vi "UUDT Engine.vi"() -> ()   [LabVIEW 2013, in "GMLAN.lvlib"]
uses:
  GMLAN.lvlib
  <vilib>/Automotive Diagnostic Command Set/Diagnostic Transport.llb/Diag Reference.ctl
  <vilib>/Automotive Diagnostic Command Set/Diagnostic Transport.llb/Transport Protocol Selector.ctl
  <vilib>/Automotive Diagnostic Command Set/Diagnostic Transport.llb/Diag CAN Frame Log.ctl
  <vilib>/xnet/xnet.llb/XNET Frame CAN.ctl
  <vilib>/xnet/xnet.llb/XNET Frame Type CAN.ctl
  UUDT Engine Connection List_Action.ctl
  UUDT Messages.ctl
  UUDT Responses.ctl
  <vilib>/xnet/xnet.llb/XNET Read (Frame CAN).vi
  <vilib>/xnet/xnet.llb/XNET Database Close (Database).vi
  <vilib>/addons/Automotive Diagnostic Command Set/NI_Automotive Diagnostic Command Set.lvlib
panel:
  in  "ADCS Ref":T1
  in  "UUDT":u32
  out "error in":errorcluster
  in  "error out":errorcluster
  in  "Database":refnum<k21>
  in  "Read":refnum<k21>
  in  "stop":bool
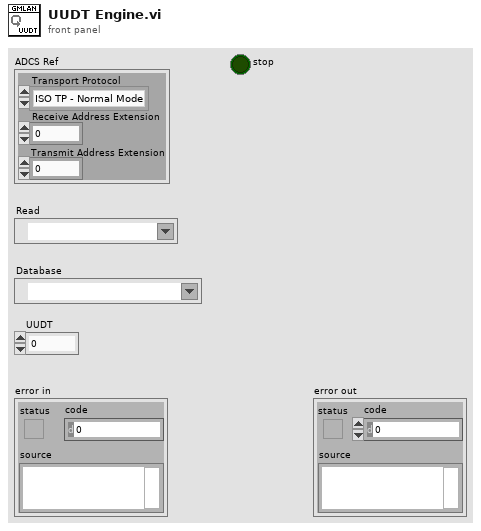
[diagram p1: front panel]
types:
  T1 = typedef "NI_Automotive Diagnostic Command Set.lvlib/Diag Reference.ctl" = cluster{"Diag CAN Handle":u32, "Transport Protocol":T2, "Receive Address Extension":u8, "Transmit Address Extension":u8, "Receive CAN Id":u32, "Transmit CAN Id":u32, "Diag CAN Queue":refnum<queue>, "Log Frames ?":bool, "My TP Address":u8, "Other TP Address":u8, "T1":u16, "T2":u16, "T3":u16, "T4":u16, "Tx SN":u8, "Block Size":u8, "Rx SN":u8, "VW TP Initialized?":bool, "Tx block no":u8, "baud rate":u32, "Interface":string, "Channel Diag CAN Handle":u32, "UDP Connection ID":refnum<k16>, "TCP Connection ID":refnum<k5>, "Target IP Addr":u32, "Source Address":u16, "Target Address":u16, "Send Header NACK?":bool, "DLL Handle":u32, "NAD":u8}
  T2 = typedef "NI_Automotive Diagnostic Command Set.lvlib/Transport Protocol Selector.ctl" = enum16{"ISO TP - Normal Mode", "ISO TP - Mixed Mode", "VW TP 2.0", "Diagnostics on IP", "ISO TP LIN"}
  T3 = typedef "XNET Frame CAN.ctl" = cluster{"timestamp":timestamp, "payload":u8[], "identifier":u32, "type":T4, "extended?":bool, "echo?":bool}
  T4 = typedef "XNET Frame Type CAN.ctl" = u8
  T5 = typedef "GMLAN.lvlib/UUDT Engine Connection List_Action.ctl" = enum8{"Initialize", "Write", "Add", "Read"}
  T6 = typedef "GMLAN.lvlib/UUDT Messages.ctl" = cluster{"UUDT Reponses":T7, "Data":T3[]}
  T7 = typedef "GMLAN.lvlib/UUDT Responses.ctl" = enum16{"DPID", "DTCStatus", "DTCReport", "ChangeDTCCount"}
  T8 = typedef "NI_Automotive Diagnostic Command Set.lvlib/Diag CAN Frame Log.ctl" = cluster{"Timestamp":dbl, "ArbitrationId":u32, "IsRemote":u8, "DataLength":u8, "Data":u8[]}
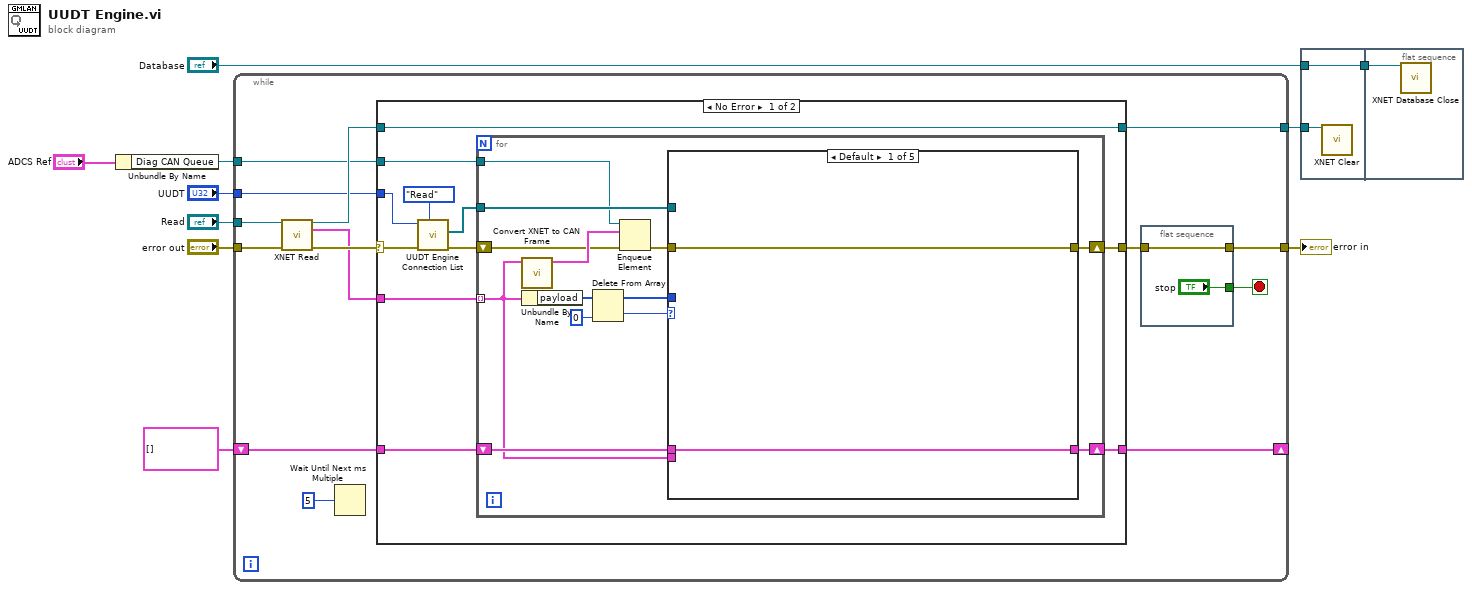
[diagram p0: block diagram]
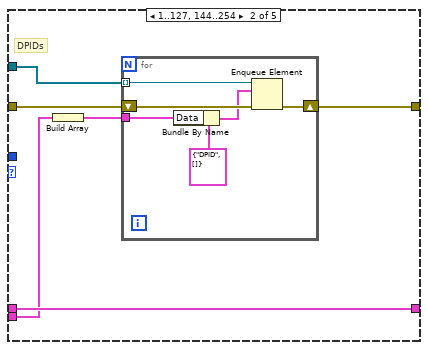
[diagram p2: hidden frame]
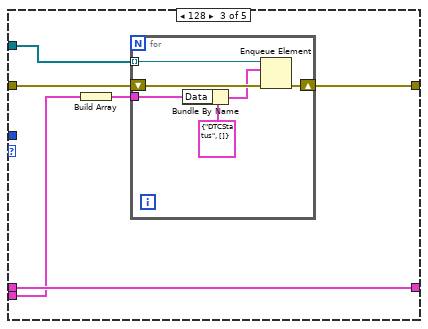
[diagram p3: hidden frame]
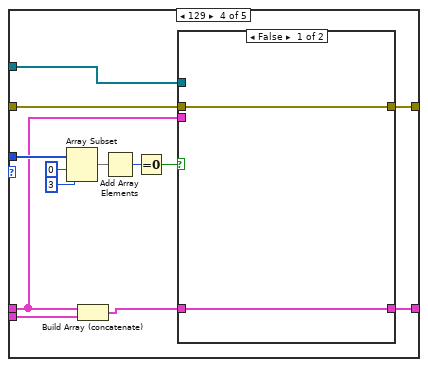
[diagram p4: hidden frame]
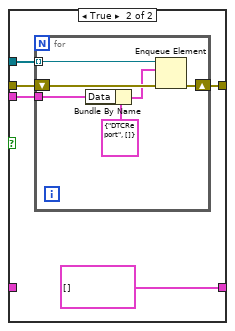
[diagram p5: hidden frame]
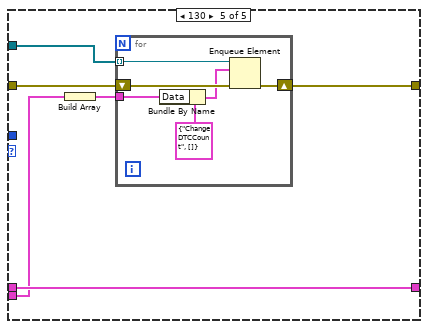
[diagram p6: hidden frame]
diagram:
  n1 = Unbundle By Name("ADCS Ref") -> ("Diag CAN Queue"=w2:refnum<queue>)
  n2 = while {
    tunnel: "error out" -> [w22]
    shift-right: [w18] -> _
    shift-left: T3[] [] ("data") -> [w19]
    tunnel: [w12] -> w4
    tunnel: "Read" -> [w23]
    tunnel: [w16] -> w9
    tunnel: "UUDT" -> [w15]
    tunnel: w2 -> [w14]
    stop <- w11 stop-if-true
    n3 = call-poly <vilib>:"XNET Read.vi"("session in"=w23, "error in (no error)"=w22) -> ("session out"=w17:refnum<k21>, "data"=w20:T3[], "error out"=w21:errorcluster)  [unwired: 10 in, 1 out]
    n4 = Wait Until Next ms Multiple(millisecond multiple=5) -> ()  [unwired: 1 out]
    n5 = case shown="No Error" w21 {
      selector: w21 -> [w31 w117]
      tunnel: w20 -> [w33 _]
      tunnel: [w35 w117] -> w13
      tunnel: w19 -> [w37 w116]
      tunnel: [w36 w116] -> w18
      tunnel: w17 -> [w34 w115]
      tunnel: [w34 w115] -> w16
      tunnel: w15 -> [w28 _]
      tunnel: w14 -> [w27 _]
      frame No Error {
        n6 = call "UUDT Engine Connection List.vi"("Action"=UUDT_Engine_Connection_List_Action."Read", "error in"=w31, "UUDT"=w28) -> ("error out"=w30:errorcluster, "Queue List"=w29:refnum<queue>[])  [unwired: 7 in]
        n7 = for {
          tunnel: w33 -> [w41] mode=indexing
          shift-right: [w48] -> w36
          shift-left: w37 -> [w49]
          shift-right: [w47] -> w35
          shift-left: w30 -> [w40]
          tunnel: w29 -> [w43]
          tunnel: w27 -> [w38]
          n8 = call "Convert XNET to CAN Frame.vi"("XNET frame"=w41) -> ("CAN Frame"=w42:T8)  [unwired: 10 in]
          n9 = Unbundle By Name(w41) -> ("payload"=w46:u8[])
          n10 = Delete From Array(array=w46, index=0) -> (deleted portion=w50:u8, array with subset deleted=w44:u8[])  [unwired: 1 in]
          n11 = Enqueue Element(queue=w38, element=w42, error in (no error)=w40) -> (error out=w39:errorcluster)  [unwired: 1 in, 2 out]
          n12 = case shown="Default" w50 {
            tunnel: w44 -> [_ _ _ w89 _]
            tunnel: w49 -> [w52 w58 w70 w81 w108]
            tunnel: w41 -> [_ w54 w66 w84 w104]
            tunnel: [w52 w58 w70 w78 w108] -> w48
            tunnel: [w51 w55 w68 w79 w106] -> w47
            tunnel: w39 -> [w51 w56 w69 w83 w107]
            tunnel: w43 -> [_ w57 w67 w80 w105]
            frame Default {
            }
            frame 1..127, 144..254 {
              # "DPIDs"
              n13 = Build Array(w54) -> (w53:T3[])
              n14 = for {
                tunnel: w57 -> [w64] mode=indexing
                shift-right: [w62] -> w55
                shift-left: w56 -> [w63]
                tunnel: w53 -> [w60]
                n15 = Bundle By Name(cluster=T6 {"UUDT Reponses"=enum."DPID", "Data"=[]} ("element"), "Data"=w60) -> (w59:T6)
                n16 = Enqueue Element(queue=w64, element=w59, error in (no error)=w63) -> (error out=w62:errorcluster)  [unwired: 1 in, 2 out]
              }
            }
            frame 128 {
              n17 = Build Array(w66) -> (w65:T3[])
              n18 = for {
                tunnel: w67 -> [w76] mode=indexing
                shift-right: [w74] -> w68
                shift-left: w69 -> [w75]
                tunnel: w65 -> [w72]
                n19 = Bundle By Name(cluster=T6 {"UUDT Reponses"=enum."DTCStatus", "Data"=[]} ("element"), "Data"=w72) -> (w71:T6)
                n20 = Enqueue Element(queue=w76, element=w71, error in (no error)=w75) -> (error out=w74:errorcluster)  [unwired: 1 in, 2 out]
              }
            }
            frame 129 {
              n21 = Array Subset(array=w89, index=0, length=3) -> (w86:u8[])
              n22 = Build Array (concatenate)(w81, w84) -> (w77:T3[])
              n23 = Add Array Elements(numeric array=w86) -> (sum=w85:u8)
              n24 = Equal To 0?(x=w85) -> (x = 0?=w82:bool)
              n25 = case shown="False" w82 {
                tunnel: w83 -> [w91 w96]
                tunnel: w81 -> [_ w95]
                tunnel: w80 -> [_ w94]
                tunnel: [w91 w93] -> w79
                tunnel: [w90 T3[] [] ("data")] -> w78
                tunnel: w77 -> [w90 _]
                frame False {
                }
                frame True {
                  n26 = for {
                    tunnel: w94 -> [w102] mode=indexing
                    shift-right: [w100] -> w93
                    shift-left: w96 -> [w101]
                    tunnel: w95 -> [w99]
                    n27 = Bundle By Name(cluster=T6 {"UUDT Reponses"=enum."DTCReport", "Data"=[]} ("element"), "Data"=w99) -> (w98:T6)
                    n28 = Enqueue Element(queue=w102, element=w98, error in (no error)=w101) -> (error out=w100:errorcluster)  [unwired: 1 in, 2 out]
                  }
                }
              }
            }
            frame 130 {
              n29 = Build Array(w104) -> (w103:T3[])
              n30 = for {
                tunnel: w105 -> [w110] mode=indexing
                shift-right: [w113] -> w106
                shift-left: w107 -> [w114]
                tunnel: w103 -> [w112]
                n31 = Bundle By Name(cluster=T6 {"UUDT Reponses"=enum."ChangeDTCCount", "Data"=[]} ("element"), "Data"=w112) -> (w111:T6)
                n32 = Enqueue Element(queue=w110, element=w111, error in (no error)=w114) -> (error out=w113:errorcluster)  [unwired: 1 in, 2 out]
              }
            }
          }
        }
      }
      frame Error {
      }
    }
    n33 = flat-sequence {
      tunnel: w13 -> [w26]
      tunnel: [w26] -> w12
      tunnel: ["stop"] -> w11
      frame #0 {
      }
    }
  }
  "error in" <- w4
  n34 = flat-sequence {
    tunnel: w9 -> [w119]
    tunnel: [w118] -> w10
    tunnel: "Database" -> [w118]
    tunnel: w10 -> [w120]
    frame #0 {
      n35 = call <vilib>:"XNET Clear.vi"("session in"=w119) -> ()  [unwired: 14 in, 1 out]
    }
    frame #1 {
      n36 = call-poly <vilib>:"XNET Database Close.vi"("database in"=w120) -> ()  [unwired: 14 in, 1 out]
    }
  }
